vi "Clean Children List.vi"(8 "error in (no error)":errorcluster, 11 "Base Tree in":refnum<class "Base Tree.lvclass">) -> (0 "error out":errorcluster, 3 "Base Tree out":refnum<class "Base Tree.lvclass">)   [LabVIEW 2017, in "Browser Core.lvlib" / "Base Tree.lvclass"]
doc: "Remove children from Node's Child list if they do not currently exist in the dictionary. Nodes do not keep track of their parents so this VI should be called after items are removed from the dictionary."
uses:
  Base Tree.lvclass
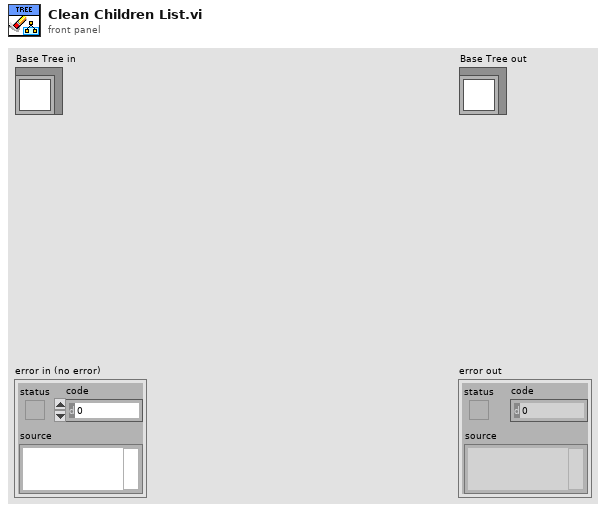
[diagram p1: front panel]
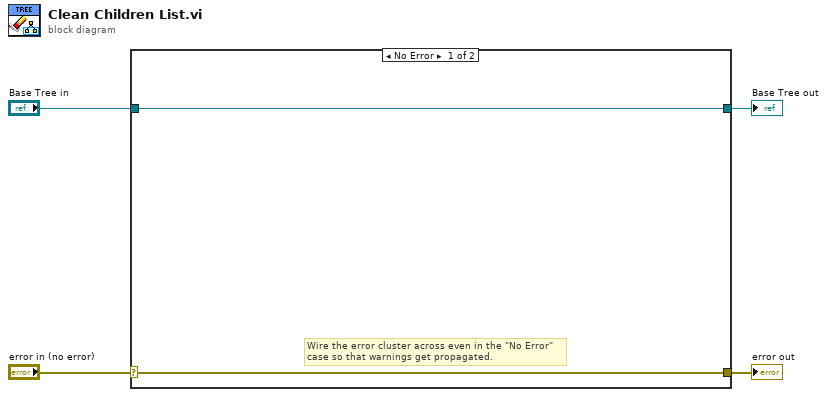
[diagram p0: block diagram]
diagram:
  n1 = case shown="No Error" "error in (no error)" {
    selector: "error in (no error)" -> [w5 w8]
    tunnel: [w5 w8] -> w3
    tunnel: [w6 w7] -> w1
    tunnel: "Base Tree in" -> [w6 w7]
    frame No Error {
      # "Wire the error cluster across even in the \"No Error\"\ncase so that warnings get propagated."
    }
    frame Error {
    }
  }
  "error out" <- w3
  "Base Tree out" <- w1
